vi "State Enter Core.vi"(8 "error in (no error)":errorcluster, 11 "B Context State in":refnum<class "B Context State.lvclass">) -> (0 "error out":errorcluster, 3 "B Context State out":refnum<class "B Context State.lvclass">)   [LabVIEW 2021, in "Context.lvlib" / "B Context State.lvclass"]
uses:
  B Context State.lvclass
  B Context State.lvclass/B Context State.ctl
  Context/Context.lvclass
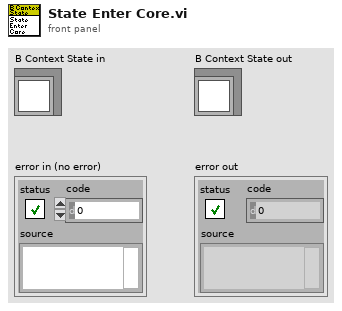
[diagram p1: front panel]
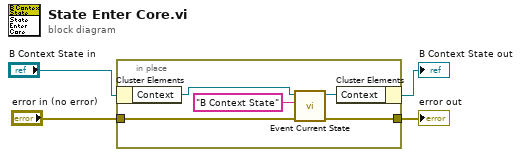
[diagram p0: block diagram]
diagram:
  n1 = in-place {
    in-place-border: "error in (no error)" -> [w7]
    in-place-border: [w6] -> w4
    n2 = in-place-cluster #1("B Context State in") -> ("Context"=w9:refnum<class "Context.lvclass">)
    n3 = call "Event Current State.vi"("error in (no error)"=w7, "Current State"="B Context State", "Context in"=w9) -> ("error out"=w6:errorcluster, "Context out"=w8:refnum<class "Context.lvclass">)  [unwired: 7 in]
    n4 = in-place-cluster #1("Context"=w8) -> (→"B Context State out":refnum<class "B Context State.lvclass">)
  }
  "error out" <- w4
